vi "Enqueue Message.vi"(6 "high priority":bool, 7 "message":T5, 8 "error in":errorcluster, 10 "data":variant, 11 "module reference in":T1) -> (0 "error out":errorcluster, 3 "module reference out":T1)   [LabVIEW 2015, in "Game.lvlib"]
uses:
  Game.lvlib
  Private TypeDefs/Messages.ctl
  Private TypeDefs/Module Reference.ctl
  Global TypeDefs/Registered Modules.ctl
  Private TypeDefs/Module Queues.ctl
  Private TypeDefs/Message Queue Element.ctl
  Private TypeDefs/Module Notifiers.ctl
  Private TypeDefs/Dummy Notifier.ctl
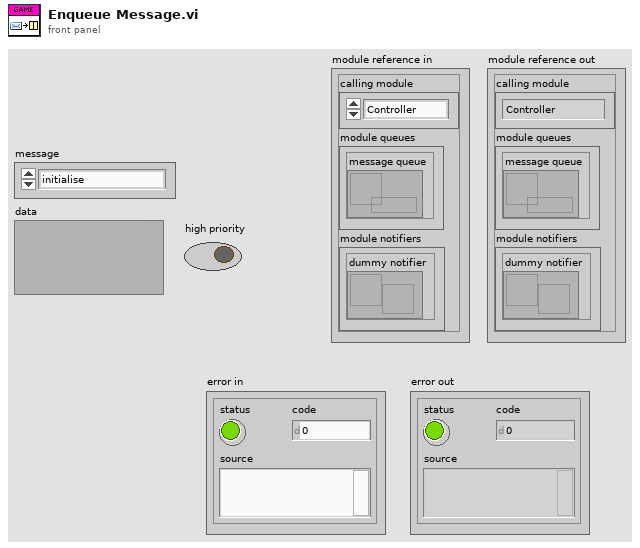
[diagram p1: front panel]
types:
  T1 = typedef "Game.lvlib/Module Reference.ctl" = cluster{"calling module":T2, "module queues":T3, "module notifiers":T4}
  T2 = typedef "Registered Modules.ctl" = enum16{"Controller", "DAQ", "Error Handler", "Game", "myPAM", "WinHost", "Logger"}
  T3 = typedef "Game.lvlib/Module Queues.ctl" = cluster{"message queue":refnum<queue>}
  T4 = typedef "Game.lvlib/Module Notifiers.ctl" = cluster{"dummy notifier":refnum<notifier>}
  T5 = typedef "Game.lvlib/Messages.ctl" = enum16{"initialise", "wait for client", "communicate", "shutdown"}
  T6 = typedef "Game.lvlib/Message Queue Element.ctl" = cluster{"source":T2, "message":T5, "data":variant}
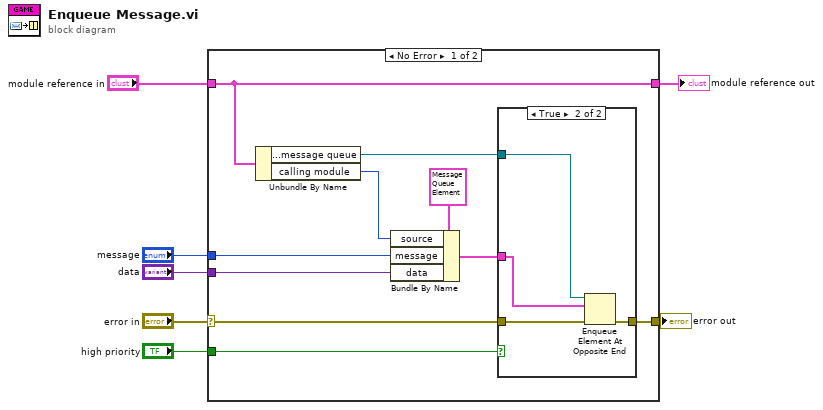
[diagram p0: block diagram]
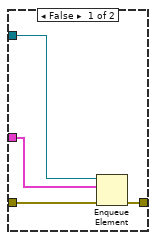
[diagram p2: hidden frame]
diagram:
  n1 = case shown="No Error" "error in" {
    selector: "error in" -> [w15 w26]
    tunnel: "data" -> [w17 _]
    tunnel: "message" -> [w16 _]
    tunnel: [w14 w26] -> w4
    tunnel: "high priority" -> [w13 _]
    tunnel: "module reference in" -> [w8 _]
    tunnel: [w8 _] -> w1
    frame No Error {
      n2 = Unbundle By Name(w8) -> ("module queues.message queue"=w10:refnum<queue>, "calling module"=w12:T2)
      n3 = Bundle By Name(cluster=T6 {"source"=enum."Controller", "message"=enum."initialise", "data"=variant} ("message queue element"), "source"=w12, "message"=w16, "data"=w17) -> (w9:T6)
      n4 = case shown="True" w13 {
        tunnel: w15 -> [w21 w25]
        tunnel: [w20 w24] -> w14
        tunnel: w10 -> [w19 w22]
        tunnel: w9 -> [w18 w23]
        frame False {
          n5 = Enqueue Element(queue=w19, element=w18, error in (no error)=w21) -> (error out=w20:errorcluster)  [unwired: 1 in, 2 out]
        }
        frame True {
          n6 = Enqueue Element At Opposite End(queue=w22, element=w23, error in (no error)=w25) -> (error out=w24:errorcluster)  [unwired: 1 in, 2 out]
        }
      }
    }
    frame Error {
    }
  }
  "error out" <- w4
  "module reference out" <- w1
